vi "sub_Loop.vi"(0 "Input parameters":T3={"Measurement type"=enum."Debug", "Sensor type"=enum."HPK_8in_256", "Identifier"="test.txt", "Open after execution?"=FALSE, "Plot after execution?"=FALSE, "Display channel"=0, "Voltage Delay (s)"=0.5, "Switch Delay (s)"=0.01, "VISA resource name source"="", "VISA resource name DMM"="", "VISA resource name LCR"="", "Compliance  Level (uA)"=10.0, "Voltage Limit (V)"=1000.0, "Data storage location"="", "Scan voltages"="", "Use source as DMM?"=FALSE, "Single channel?"=FALSE, "LCR signal frequenzy (Hz)"=10.0, "DMM device"=enum."Keithley2001", "Sampling number"=1, "Use env. sensors on"=enum."Sensirion sht1x/7x", "Switchboard Handle"=0, "Use Switchboard"=FALSE, "LCR signal voltage (V)"=10000.0, "Repeat"=1, "Test Run Limit (nA)"=10.0, "Scan voltages IV"="", "Scan voltages CV"="", "Hex pad numbers?"=FALSE, "Set measurement type"=enum."Debug"} {"Voltage Limit (V)" format="%#_13g"; "Voltage Delay (s)" format="%#_13g"; "Switch Delay (s)" format="%#_13g"}, 1 "Current channel":refnum<vi>, 2 "Current voltage":refnum<vi>, 3 "Elapsed time":refnum<vi>, 5 "Dynamic data":T2, 8 "Channels":refnum<vi>, 9 "Stop":refnum<vi>, 10 "Single channel":refnum<vi>, 11 "error in (no error)":errorcluster, 12 "Environmental data":T1, 14 "Estimated remaining time":refnum<vi>) -> (4 "Input parameters":T3={"Measurement type"=enum."Debug", "Sensor type"=enum."HPK_8in_256", "Identifier"="test.txt", "Open after execution?"=FALSE, "Plot after execution?"=FALSE, "Display channel"=0, "Voltage Delay (s)"=0.5, "Switch Delay (s)"=0.01, "VISA resource name source"="", "VISA resource name DMM"="", "VISA resource name LCR"="", "Compliance  Level (uA)"=10.0, "Voltage Limit (V)"=1000.0, "Data storage location"="", "Scan voltages"="", "Use source as DMM?"=FALSE, "Single channel?"=FALSE, "LCR signal frequenzy (Hz)"=10.0, "DMM device"=enum."Keithley2001", "Sampling number"=1, "Use env. sensors on"=enum."Sensirion sht1x/7x", "Switchboard Handle"=0, "Use Switchboard"=FALSE, "LCR signal voltage (V)"=10000.0, "Repeat"=1, "Test Run Limit (nA)"=10.0, "Scan voltages IV"="", "Scan voltages CV"="", "Hex pad numbers?"=FALSE, "Set measurement type"=enum."Debug"} {"Voltage Limit (V)" format="%#_13g"; "Voltage Delay (s)" format="%#_13g"; "Switch Delay (s)" format="%#_13g"}, 6 "Dynamic data":T2, 15 "error out":errorcluster)   [LabVIEW 2016]
uses:
  Input_parameters.ctl
  Dynamic_data.ctl
  <extravilib>/ChannelInstances/Tag-t'Env_data.ctl'/))Channel.ctl
  Env_data.ctl
  <extravilib>/ChannelInstances/Tag-t'Env_data.ctl'/Read With Abort.vi
  <extravilib>/ChannelInstances/Tag-t'Env_data.ctl'/Endpoint.vi
  <extravilib>/ChannelInstances/Tag-t'Env_data.ctl'.lvlib
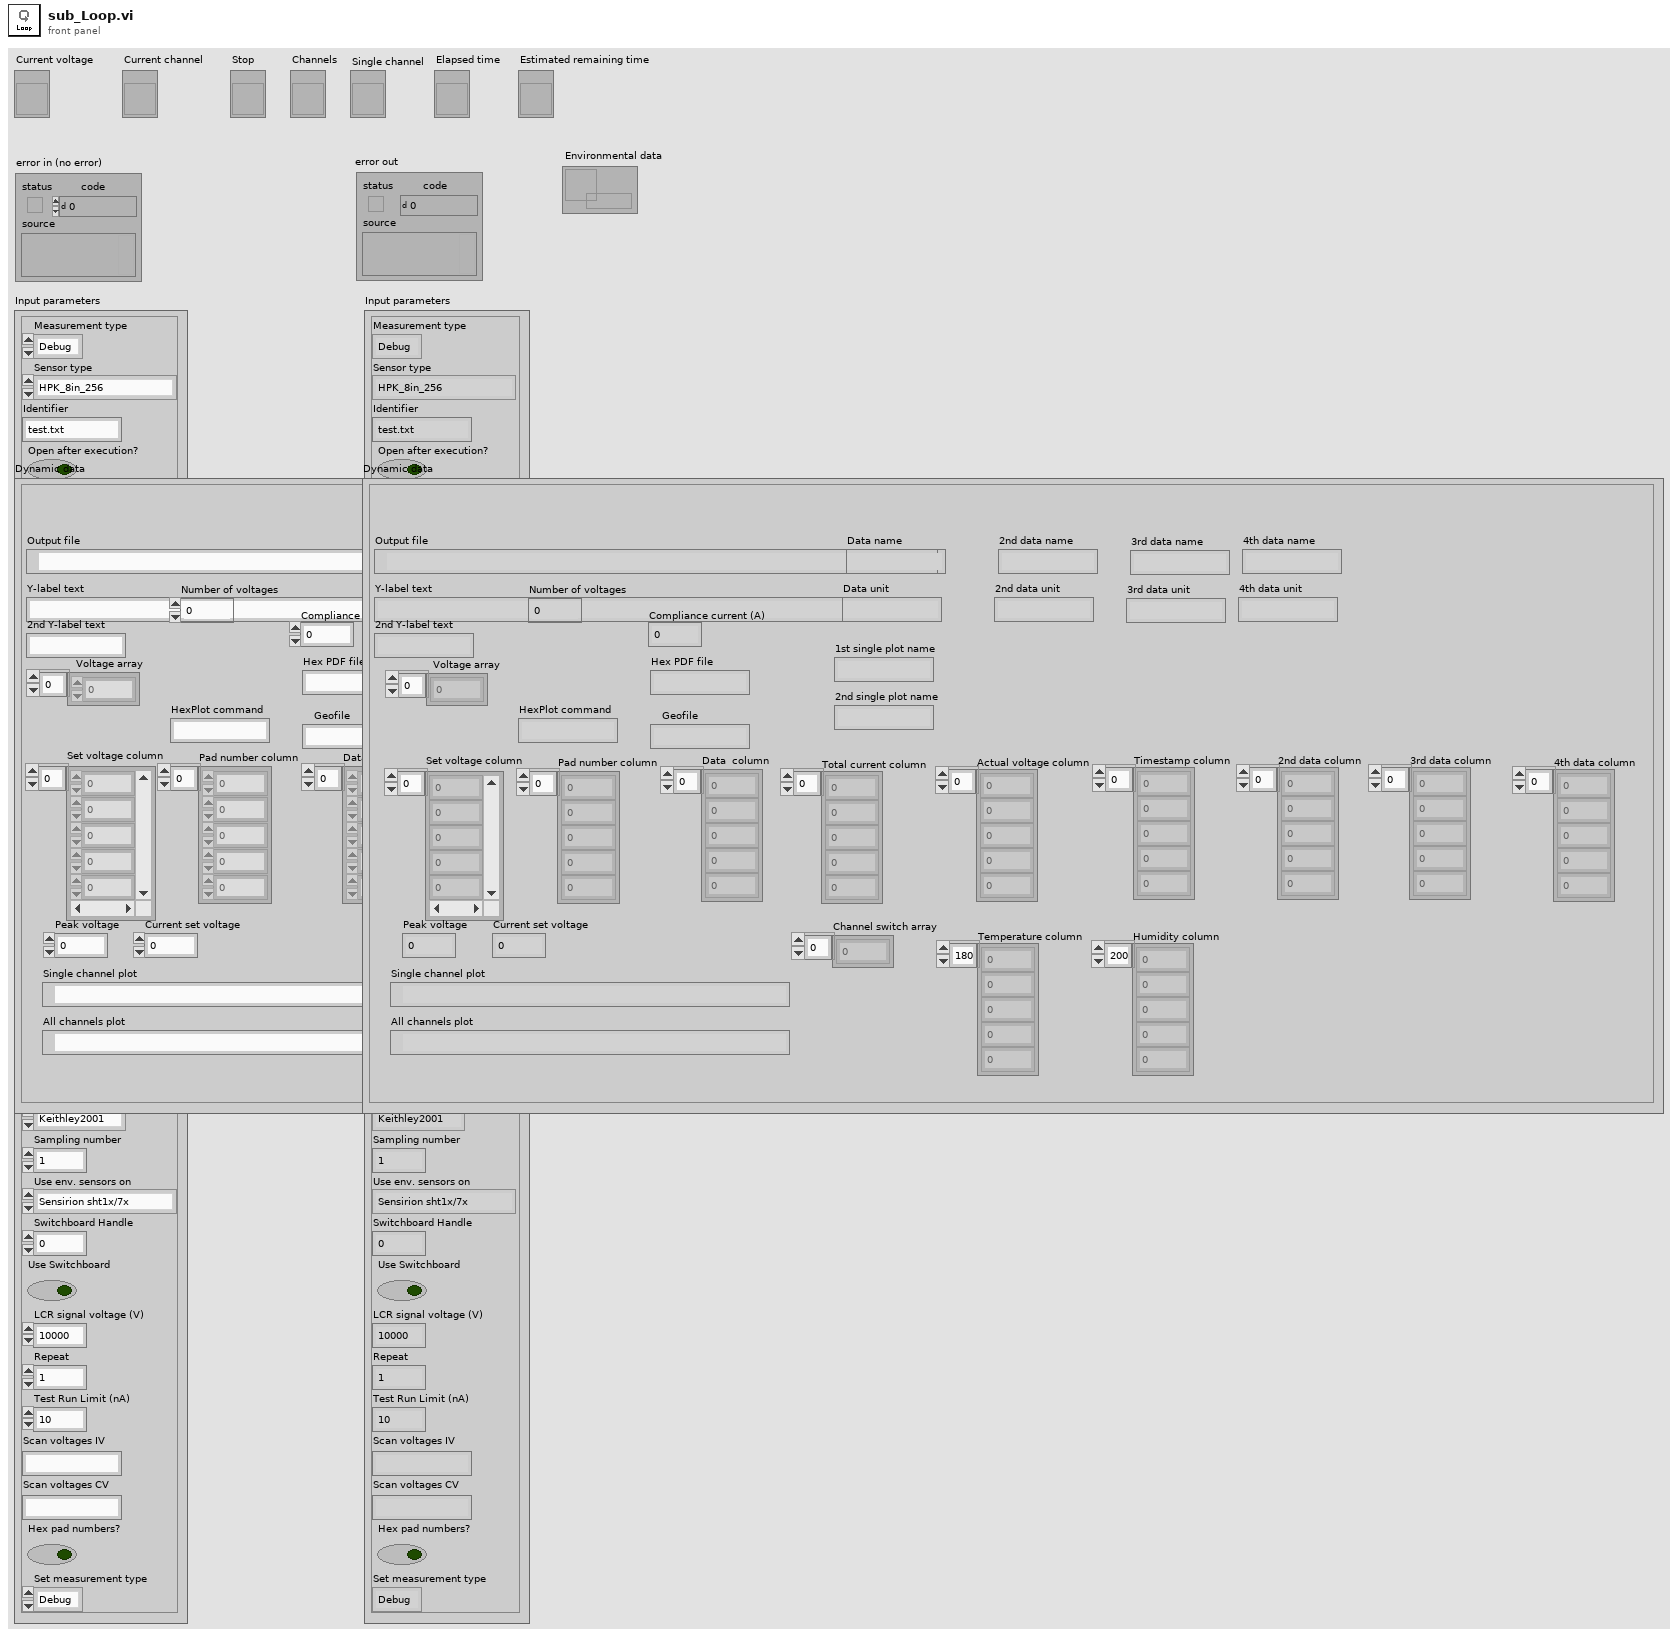
[diagram p1: front panel]
types:
  T1 = typedef "Tag-t'Env_data.ctl'.lvlib/))Channel.ctl" = refnum<queue>
  T2 = typedef "Dynamic_data.ctl" = cluster{"Output file":path, "Y-label text":string, "Current set voltage":dbl, "Set voltage column":dbl[], "Pad number column":dbl[], "Data  column":dbl[], "Number of voltages":i32, "Compliance current (A)":dbl, "Geofile":string, "Peak voltage":dbl, "Hex PDF file":string, "Voltage array":dbl[], "Total current column":dbl[], "Timestamp column":dbl[], "Data name":string, "Data unit":string, "2nd data column":dbl[], "2nd data name":string, "2nd data unit":string, "3rd data column":dbl[], "4th data column":dbl[], "3rd data name":string, "3rd data unit":string, "4th data name":string, "4th data unit":string, "Actual voltage column":dbl[], "2nd Y-label text":string, "Single channel plot":path, "Temperature column":dbl[], "Humidity column":dbl[], "Channel switch array":i32[], "1st single plot name":string, "2nd single plot name":string, "All channels plot":path, "HexPlot command":string}
  T3 = typedef "Input_parameters.ctl" = cluster{"Measurement type":enum16{"IV", "CV", "Debug", "Test"}, "Sensor type":enum16{"HPK_6in_135", "HPK_8in_256", "INF_8in_256", "Diode", "HPK_6in_256", "Test capacitances", "Full matrix"}, "Identifier":string, "Open after execution?":bool, "Plot after execution?":bool, "Display channel":i32, "Voltage Delay (s)":dbl, "Switch Delay (s)":dbl, "VISA resource name source":refnum<visa-resource-name>, "VISA resource name DMM":refnum<visa-resource-name>, "VISA resource name LCR":refnum<visa-resource-name>, "Compliance  Level (uA)":dbl, "Voltage Limit (V)":dbl, "Data storage location":string, "Scan voltages":string, "Use source as DMM?":bool, "Single channel?":bool, "LCR signal frequenzy (Hz)":dbl, "DMM device":enum16{"Keithley2001", "Keithley2450", "Keithley2410", "Keithley6487"}, "Sampling number":i32, "Use env. sensors on":enum16{"Sensirion sht1x/7x", "Switch Matrix", "Probecard"}, "Switchboard Handle":u32, "Use Switchboard":bool, "LCR signal voltage (V)":dbl, "Repeat":i32, "Test Run Limit (nA)":dbl, "Scan voltages IV":string, "Scan voltages CV":string, "Hex pad numbers?":bool, "Set measurement type":enum16{"IV", "CV", "Debug", "Test", "IV+CV"}}
  T4 = enum16{"Sensirion sht1x/7x", "Switch Matrix", "Probecard"}
  T5 = typedef "Env_data.ctl" = cluster{"Temp. Sensirion":dbl, "Hum. Sensirion":dbl, "Temp. Switch Matrix":dbl, "Hum. Switch Matrix":dbl, "Temp. Probecard":dbl, "Hum. Probecard":dbl}
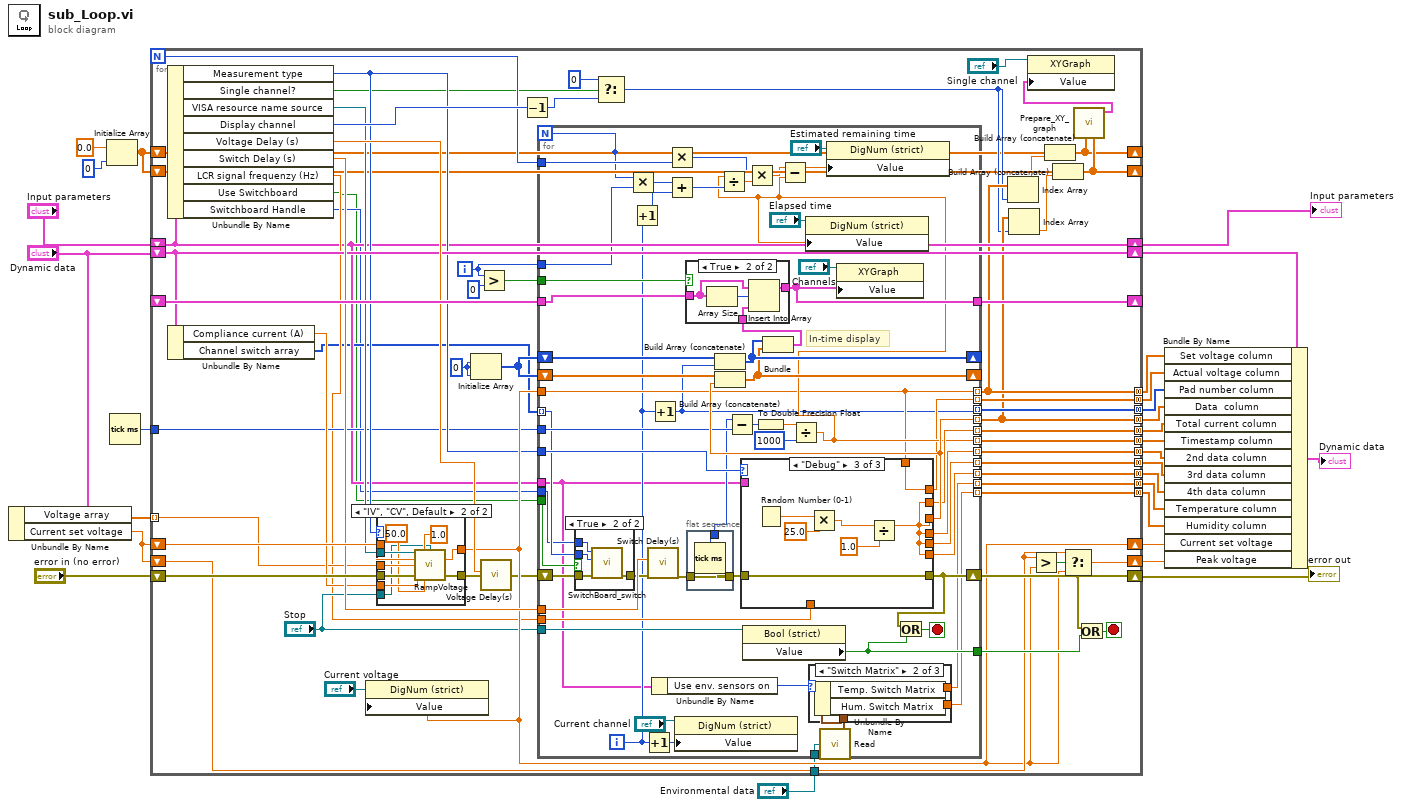
[diagram p0: block diagram]
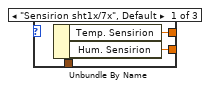
[diagram p3: hidden frame]
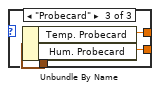
[diagram p4: hidden frame]
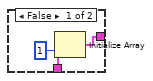
[diagram p6: hidden frame]
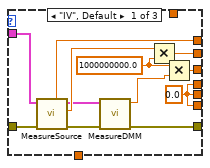
[diagram p7: hidden frame]
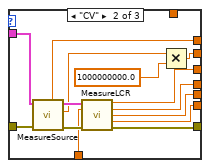
[diagram p8: hidden frame]
diagram:
  n1 = Unbundle By Name("Dynamic data") -> ("Voltage array"=w27:dbl[], "Current set voltage"=w16:dbl)
  n2 = Initialize Array(0.0 ("Secondary Parameter"), 0 ("dimension size")) -> (w1:dbl[])
  n3 = Tick Count (ms)() -> (millisecond timer value=w17:u32)
  n4 = for {
    N -> [w54]
    tunnel: w27 -> [w63] mode=indexing
    tunnel: [w38] -> w26 mode=concatenating
    tunnel: [w37] -> w24 mode=concatenating
    tunnel: [w85] -> w25 mode=concatenating
    shift-right: [w76] -> w18
    shift-left: "error in (no error)" -> [w84]
    shift-right: [w81] -> _
    shift-left: _ -> [w80]
    shift-right: [w65] -> w7
    shift-left: w16 -> [w75]
    shift-right: [w50] -> w20
    shift-left: "Input parameters" -> [w50]
    shift-right: [w72] -> w23
    shift-left: "Dynamic data" -> [w72]
    tunnel: w17 -> [w58]
    shift-right: [w67] -> w8
    shift-left: w16 -> [w66]
    tunnel: [w59] -> w14 mode=concatenating
    tunnel: [w57] -> w13 mode=concatenating
    tunnel: [w56] -> w12 mode=concatenating
    tunnel: [w52] -> w11 mode=concatenating
    tunnel: [w51] -> w10 mode=concatenating
    tunnel: [w49] -> w9 mode=concatenating
    tunnel: [w48] -> w6 mode=concatenating
    tunnel: [w47] -> w5 mode=concatenating
    tunnel: "Environmental data" -> [w46]
    shift-right: [w30] -> _
    shift-left: w1 -> [w35]
    shift-right: [w31] -> _
    shift-left: w1 -> [w34]
    i -> [w55]
    stop <- w77 stop-if-true
    w45 = 0 ("dimension size")
    n5 = Unbundle By Name(w50) -> ("Measurement type"=w61:enum16{"IV", "CV", "Debug", "Test"}, "Single channel?"=w42:bool, "VISA resource name source"=w62:refnum<visa-resource-name>, "Display channel"=w69:i32, "Voltage Delay (s)"=w74:dbl, "Switch Delay (s)"=w73:dbl, "LCR signal frequenzy (Hz)"=w53:dbl, "Use Switchboard"=w39:bool, "Switchboard Handle"=w40:u32)
    n6 = Unbundle By Name(w72) -> ("Compliance current (A)"=w71:dbl, "Channel switch array"=w44:i32[])
    n7 = case shown="\"IV\", \"CV\", Default" w61 {
      tunnel: w62 -> [_ w96]
      tunnel: w63 -> [w87 w95]
      tunnel: w84 -> [w88 w97]
      tunnel: [w88 w98] -> w83
      tunnel: w71 -> [_ w93]
      tunnel: w75 -> [_ w94]
      tunnel: [w87 w90] -> w65
      tunnel: "Stop" -> [_ w89]
      frame "Debug" {
      }
      frame "IV", "CV", Default {
        n8 = call "RampVoltage.vi"("VISA resource name"=w96, "Delay (s)"=1.0, "Stop"=w89, "Current voltage (V)"=w94, "Target voltage (V)"=w95, "Compliance Current (A)"=w93, "error in (no error)"=w97, "Step size (V)"=50.0) -> ("Current voltage out (V)"=w90:dbl, "error out"=w98:errorcluster)  [unwired: 5 in, 1 out]
      }
    }
    n9 = property class="DigNum (strict)"(reference="Current voltage", "Value"=w65) -> ()  [unwired: 1 in, 2 out]
    n10 = Initialize Array(w45, w45) -> (w79:i32[])
    n11 = Greater?(x=w55, y=0) -> (0:w82:bool)
    n12 = call "Voltage Delay(s)"("error in (no error)"=w83, "Delay Time (s)"=w74) -> ("error out"=w60:errorcluster)  [unwired: 9 in]
    n13 = Decrement(x=w69) -> (x-1=w43:i32)
    n14 = for {
      N -> [w122]
      tunnel: w44 -> [w105] mode=indexing
      tunnel: [w99] -> w85 mode=indexing
      tunnel: [w154] -> w37 mode=indexing
      tunnel: w65 -> [w113]
      tunnel: [w113] -> w38 mode=indexing
      tunnel: w61 -> [w156]
      shift-right: [w147] -> w76
      shift-left: w60 -> [w107]
      shift-right: [w152] -> _
      shift-left: w79 -> [w155]
      shift-right: [w151] -> _
      shift-left: w79 -> [w153]
      tunnel: w82 -> [w150]
      tunnel: w80 -> [w149]
      tunnel: [w141] -> w81
      tunnel: [w143] -> w78
      tunnel: w73 -> [w145]
      tunnel: "Stop" -> [w140]
      tunnel: [w138] -> w59 mode=indexing
      tunnel: w58 -> [w137]
      tunnel: [w117] -> w57 mode=indexing
      tunnel: [w134] -> w56 mode=indexing
      tunnel: w55 -> [w123]
      tunnel: w54 -> [w129]
      tunnel: w53 -> [w112]
      tunnel: [w116] -> w52 mode=indexing
      tunnel: [w115] -> w51 mode=indexing
      tunnel: w50 -> [w101]
      tunnel: [w114] -> w49 mode=indexing
      tunnel: [w110] -> w48 mode=indexing
      tunnel: [w109] -> w47 mode=indexing
      tunnel: w46 -> [w108]
      tunnel: w40 -> [w104]
      tunnel: w39 -> [w103]
      i -> [w102]
      stop <- w146 stop-if-true
      # "In-time display"
      n15 = case shown="True" w103 {
        tunnel: w107 -> [w166 w170]
        tunnel: [w166 w169] -> w106
        tunnel: w105 -> [_ w168]
        tunnel: w104 -> [_ w167]
        frame False {
        }
        frame True {
          n16 = call "SwitchBoard_switch.vi"("error in"=w170, "Channel"=w168, "Handle"=w167) -> ("error out"=w169:errorcluster)  [unwired: 7 in, 1 out]
        }
      }
      n17 = Multiply(x=w122, y=w123) -> (x*y=w124:i32)
      n18 = Increment(x=w102) -> (x+1=w121:i32)
      n19 = Increment(x=w102) -> (x+1=w139:i32)
      n20 = call "Switch Delay(s)"("error in (no error)"=w106, "Delay Time (s)"=w145) -> ("error out"=w132:errorcluster)  [unwired: 9 in]
      n21 = Increment(x=w102) -> (x+1=w99:i32)
      n22 = Unbundle By Name(w101) -> ("Use env. sensors on"=w100:T4)
      n23 = Multiply(x=w122, y=w129) -> (x*y=w126:i32)
      n24 = Add(x=w124, y=w121) -> (x+y=w128:i32)
      n25 = property on="Property Node" class="DigNum (strict)"(reference="Current channel", "Value"=w139) -> ()  [unwired: 1 in, 2 out]
      n26 = flat-sequence {
        tunnel: [w172] -> w133
        tunnel: w132 -> [w171]
        tunnel: [w171] -> w131
        frame #0 {
          n27 = Tick Count (ms)() -> (millisecond timer value=w172:u32)
        }
      }
      n28 = Build Array (concatenate)(w155, w99) -> (w152:i32[])
      n29 = Subtract(x=w133, y=w137) -> (x-y=w135:u32)
      n30 = case shown="\"Debug\"" w156 {
        tunnel: [w189 w195 w209] -> w154
        tunnel: w131 -> [w185 w203 w212]
        tunnel: [w191 w196 w212] -> w147
        tunnel: [w188 w205 w209] -> w138
        tunnel: [w186 w192 w209] -> w134
        tunnel: [w186 w193 w209] -> w116
        tunnel: [w186 w194 w209] -> w115
        tunnel: w101 -> [w183 w201 _]
        tunnel: [w182 w202 w208] -> w114
        tunnel: w113 -> [_ _ w208]
        tunnel: w112 -> [_ w197 _]
        frame "IV", Default {
          w186 = 0.0 ("Secondary Parameter")
          w187 = 1000000000.0 ("x")
          n31 = call "MeasureSource.vi"("error in (no error)"=w185, "Input parameters"=w183) -> ("error out"=w184:errorcluster, "Total current"=w181:dbl, "Input parameters"=w180:T3, "Actual voltage"=w182:dbl)  [unwired: 6 in]
          n32 = call "MeasureDMM.vi"("error in (no error)"=w184, "Input parameters"=w180) -> ("error out"=w191:errorcluster, "Result"=w190:dbl)  [unwired: 8 in]
          n33 = Multiply(x=w181, y=w187) -> (x*y=w188:dbl)
          n34 = Multiply(x=w187, y=w190) -> (x*y=w189:dbl)
        }
        frame "CV" {
          n35 = call "MeasureSource.vi"("error in (no error)"=w203, "Input parameters"=w201) -> ("error out"=w198:errorcluster, "Total current"=w199:dbl, "Input parameters"=w200:T3, "Actual voltage"=w202:dbl)  [unwired: 6 in]
          n36 = call "MeasureLCR.vi"("Input parameters"=w200, "Frequency (Hz)"=w197, "error in (no error)"=w198) -> ("Cp [pF]"=w195:dbl, "Cs [pF]"=w192:dbl, "Z (impedance)"=w193:dbl, "Theta (Phase)"=w194:dbl, "error out"=w196:errorcluster)  [unwired: 4 in, 4 out]
          n37 = Multiply(x=w199, y=1000000000.0 ("x")) -> (x*y=w205:dbl)
        }
        frame "Debug" {
          n38 = Random Number (0-1)() -> (number: 0 to 1=w207:dbl)
          n39 = Multiply(x=w207, y=25.0 ("x")) -> (x*y=w206:dbl)
          n40 = Divide(x=w206, y=1.0) -> (x/y=w209:dbl)
        }
      }
      n41 = Build Array (concatenate)(w153, w154) -> (w151:dbl[])
      n42 = property class="Bool (strict)"(reference=w140) -> ("Value"=w143:bool)  [unwired: 1 in, 2 out]
      n43 = To Double Precision Float(number=w135) -> (double precision float=w119:dbl)
      n44 = Bundle(w152, w151) -> (w148:cluster{i32[], dbl[]})  [unwired: 1 out]
      n45 = case shown="True" w150 {
        tunnel: w149 -> [_ w178]
        tunnel: [w173 w177] -> w141
        tunnel: w148 -> [w174 w176]
        frame False {
          n46 = Initialize Array(w174, 1 ("dimension size")) -> (w173:cluster{i32[], dbl[]}[])
        }
        frame True {
          n47 = Array Size(array=w178) -> (size(s)=w179:i32)
          n48 = Insert Into Array(array=w178, index=w179, new element=w176) -> (w177:cluster{i32[], dbl[]}[])
        }
      }
      n49 = Divide(x=w119, y=u32 1000) -> (x/y=w117:dbl)
      n50 = Divide(x=w117, y=w128) -> (x/y=w127:dbl)
      n51 = Multiply(x=w126, y=w127) -> (x*y=w125:dbl)
      n52 = Subtract(x=w125, y=w117) -> (x-y=w120:dbl)
      n53 = property class="DigNum (strict)"(reference="Elapsed time", "Value"=w117) -> ()  [unwired: 1 in, 2 out]
      n54 = call <extravilib>:"Read.vi"("channel"=w108) -> ("element"=w111:T5)  [unwired: 1 in, 1 out]
      n55 = case shown="\"Switch Matrix\"" w100 {
        tunnel: w111 -> [w159 w162 w165]
        tunnel: [w158 w160 w163] -> w110
        tunnel: [w157 w161 w164] -> w109
        frame "Sensirion sht1x/7x", Default {
          n56 = Unbundle By Name(w159) -> ("Temp. Sensirion"=w158:dbl, "Hum. Sensirion"=w157:dbl)
        }
        frame "Switch Matrix" {
          n57 = Unbundle By Name(w162) -> ("Temp. Switch Matrix"=w160:dbl, "Hum. Switch Matrix"=w161:dbl)
        }
        frame "Probecard" {
          n58 = Unbundle By Name(w165) -> ("Temp. Probecard"=w163:dbl, "Hum. Probecard"=w164:dbl)
        }
      }
      n59 = property class="DigNum (strict)"(reference="Estimated remaining time", "Value"=w120) -> ()  [unwired: 1 in, 2 out]
      n60 = property class="XYGraph"(reference="Channels", "Value"=w141) -> ()  [unwired: 1 in, 2 out]
      n61 = Or(x=w147, y=w143) -> (x .or. y?=w146:bool)
    }
    n62 = Select(t=0, s=w42, f=w43) -> (s? t:f=w36:i32)
    n63 = Index Array(array=w38, index=w36) -> (element=w33:dbl)
    n64 = Index Array(array=w37, index=w36) -> (element=w32:dbl)
    n65 = Greater?(x=w66, y=w65) -> (0:w68:bool)
    n66 = Build Array (concatenate)(w35, w33) -> (w30:dbl[])
    n67 = Build Array (concatenate)(w34, w32) -> (w31:dbl[])
    n68 = Select(t=w66, s=w68, f=w65) -> (s? t:f=w67:dbl)
    n69 = call "Prepare_XY_graph.vi"("Y array"=w31, "X array"=w30) -> ("XY Graph"=w29:cluster{"X array":dbl[], "Y array":dbl[]}[])  [unwired: 9 in]
    n70 = property class="XYGraph"(reference="Single channel", "Value"=w29) -> ()  [unwired: 1 in, 2 out]
    n71 = Or(x=w76, y=w78) -> (x .or. y?=w77:bool)
  }
  "error out" <- w18
  "Input parameters" <- w20
  n72 = Bundle By Name(cluster=w23, "Set voltage column"=w26, "Actual voltage column"=w9, "Pad number column"=w25, "Data  column"=w24, "Total current column"=w14, "Timestamp column"=w13, "2nd data column"=w12, "3rd data column"=w11, "4th data column"=w10, "Temperature column"=w6, "Humidity column"=w5, "Current set voltage"=w7, "Peak voltage"=w8) -> (→"Dynamic data":T2)
